vi "MoveDistance.vi"(6 "reinitialize? (F)":bool, 9 "Distance From Target":dbl) -> (1 "Done?":bool)   [LabVIEW 2013]
uses:
  <vilib>/addons/control/pid/pid.llb/PID (DBL).vi
  <vilib>/Rock Robotics/WPI/RobotDrive/WPI_RobotDriveGetSetRefNum.vi
  <vilib>/addons/control/pid/NI_PID_pid.lvlib
panel:
  in  "Adjustment Variable":dbl=0.72
  in  "PID Gains Distance":T1={"proportional gain (Kc)"=1.0, "integral time (Ti, min)"=0.01, "derivative time (Td, min)"=0.0} {"derivative time (Td, min)" format="%.3f"; "integral time (Ti, min)" format="%.3f"; "proportional gain (Kc)" format="%.3f"}
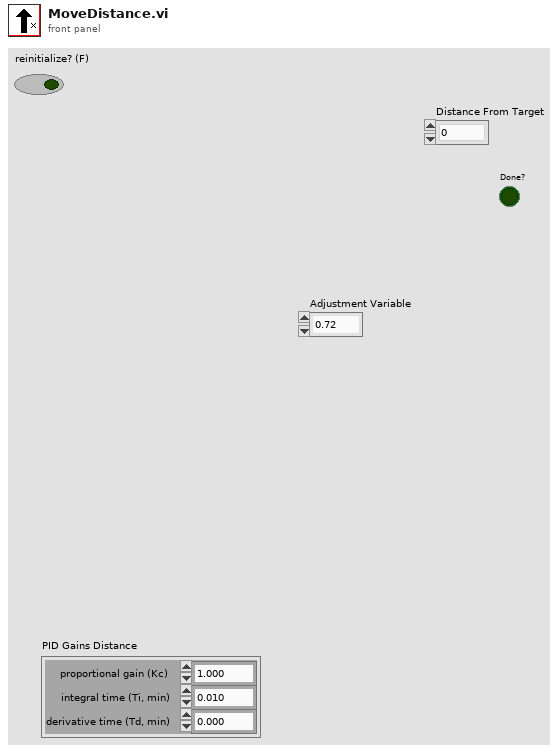
[diagram p1: front panel]
types:
  T1 = cluster{"proportional gain (Kc)":dbl, "integral time (Ti, min)":dbl, "derivative time (Td, min)":dbl}
  T2 = typedef "WPI_EncoderDevRef.ctl" = cluster{"DevStatus":errorcluster, "EncoderIndex":T3, "CounterIndex":T4, "DistancePerCount":dbl, "Decoding Type":T5}
  T3 = typedef "FPGA_EncoderIdx.ctl" = enum8{"Enc 0", "Enc 1", "Enc 2", "Enc 3", "Invalid"}
  T4 = typedef "FPGA_CounterCtrSystemIndex.ctl" = enum8{"Ctr 0", "Ctr 1", "Ctr 2", "Ctr 3", "Ctr 4", "Ctr 5", "Ctr 6", "Ctr 7", "Invalid"}
  T5 = typedef "WPI_EncoderType.ctl" = enum16{"1x", "2x", "4x"}
  T6 = typedef "WPI_RobotDriveDevRef.ctl" = cluster{"DevStatus":errorcluster, "Motors[]":T7[], "Square Inputs":bool, "Max Output":dbl, "Isochronous":bool}
  T7 = typedef "WPI_MotorControlDeviceRef.ctl" = cluster{"DeviceStatus":errorcluster, "Type":enum16{"PWM", "CAN"}, "PWM":cluster{"Digital Module":T8, "PWM Channel":T9, "DeadBand":T10}, "CAN":cluster{"Device Number":u8, "Control Mode":T11, "Semaphore":T12, "Max Vout":dbl}, "Invert":bool, "TransformRef":T13, "InvTransformRef":T13}
  T8 = typedef "FPGA_TypedefDigitalModule.ctl" = enum16{"Digital Module 1", "Digital Module 2"}
  T9 = typedef "FPGA_DIOPWMChannel.ctl" = enum8{"PWM 1", "PWM 2", "PWM 3", "PWM 4", "PWM 5", "PWM 6", "PWM 7", "PWM 8", "PWM 9", "PWM 10", "Invalid"}
  T10 = typedef "WPI_PWMDeadband.ctl" = cluster{"Name":string, "maxPositivePwm":i32, "minPositivePwm":i32, "centerPwm":i32, "maxNegativePwm":i32, "minNegativePwm":i32, "angularRange":u16}
  T11 = typedef "WPI_CANJaguar_ControlMode.ctl" = enum8{"Percent VBus", "Current", "Speed", "Position", "Voltage"}
  T12 = typedef "Semaphore RefNum" = refnum<k1>
  T13 = typedef "WPI_PWMTransform_ConPane.ctl" = refnum<vi>
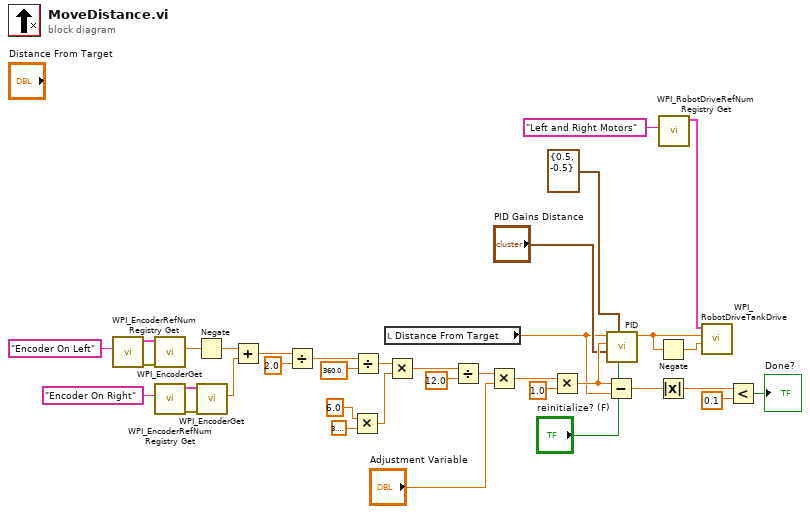
[diagram p0: block diagram]
diagram:
  n1 = call <vilib>:"WPI_EncoderRefNum Registry Get.vi"("refnum name"="Encoder On Left") -> ("error out"=w16:errorcluster, "EncoderDevRef"=w17:T2)  [unwired: 9 in]
  n2 = call <vilib>:"WPI_EncoderGet.vi"("error in (no error)"=w16, "EncoderDevRef"=w17) -> ("Distance"=w10:dbl)  [unwired: 4 in, 5 out]
  n3 = call <vilib>:"WPI_EncoderRefNum Registry Get.vi"("refnum name"="Encoder On Right") -> ("error out"=w18:errorcluster, "EncoderDevRef"=w19:T2)  [unwired: 9 in]
  n4 = Negate(x=w10) -> (-x=w9:dbl)
  n5 = call <vilib>:"WPI_EncoderGet.vi"("error in (no error)"=w18, "EncoderDevRef"=w19) -> ("Distance"=w22:dbl)  [unwired: 4 in, 5 out]
  n6 = Add(x=w9, y=w22) -> (x+y=w23:dbl)
  n7 = Divide(x=w23, y=2.0) -> (x/y=w27:dbl)
  n8 = Multiply(x=6.0, y=3.141592653589793) -> (x*y=w30:dbl)
  n9 = Divide(x=w27, y=360.0) -> (x/y=w29:dbl)
  n10 = local read "Distance From Target"() -> (w2:dbl)
  n11 = Multiply(x=w29, y=w30) -> (x*y=w31:dbl)
  n12 = Divide(x=w31, y=12.0) -> (x/y=w13:dbl)
  n13 = Multiply(x=w13, y="Adjustment Variable") -> (x*y=w12:dbl)
  n14 = Multiply(x=w12, y=1.0) -> (x*y=w8:dbl)
  n15 = Subtract(x=w8, y=w2) -> (x-y=w34:dbl)
  n16 = call-poly <vilib>:"PID.vi"("reinitialize? (F)"="reinitialize? (F)", "output range"=cluster{"output high":dbl, "output low":dbl} {"output high"=0.5, "output low"=-0.5}, "PID gains"="PID Gains Distance", "process variable"=w8, "setpoint"=w2) -> ("output"=w14:dbl)  [unwired: 5 in, 1 out]
  n17 = Negate(x=w14) -> (-x=w4:dbl)
  n18 = Absolute Value(x=w34) -> (abs(x)=w35:dbl)
  n19 = call <vilib>:"WPI_RobotDriveRefNum Registry Get.vi"("refnum name"="Left and Right Motors") -> ("RobotDriveDevRef"=w3:T6)  [unwired: 9 in, 1 out]
  n20 = call <vilib>:"WPI_RobotDriveTankDrive.vi"("Right axis value"=w4, "Left axis value"=w14, "RobotDriveDevRef"=w3) -> ()  [unwired: 6 in, 3 out]
  n21 = Less?(x=w35, y=0.1) -> (x < y?=→"Done?":bool)
